vi "Autonomous Independent.vi"(5 "Servo Positions":T1, 7 "Auton Array":dbl[][](array[numeric])) -> (3 "LED ms toggle rate":u32=500)   [LabVIEW 2013]
doc: "This VI is called when autonomous begins, and will automatically be terminated when autonomous ends. You can carry out timed or sensor driven robot movement independently without needing to return to the caller."
uses:
  <vilib>/Rock Robotics/WPI/Relay/WPI_RelayValue.ctl
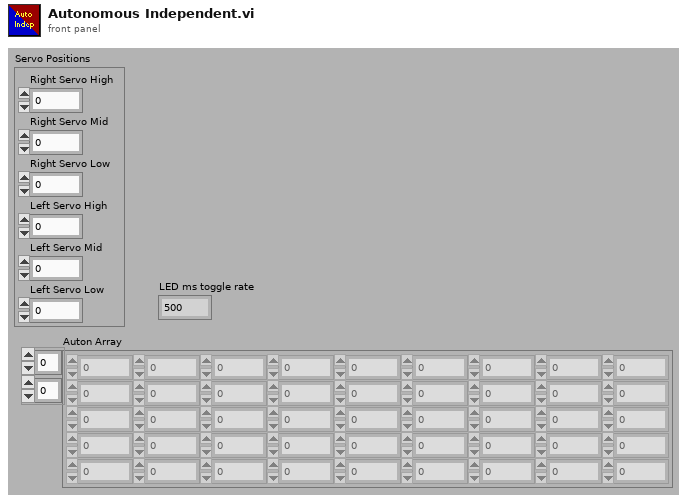
[diagram p1: front panel]
types:
  T1 = cluster{"Right Servo High":dbl, "Right Servo Mid":dbl, "Right Servo Low":dbl, "Left Servo High":dbl, "Left Servo Mid":dbl, "Left Servo Low":dbl}
  T2 = typedef "WPI_EncoderDevRef.ctl" = cluster{"DevStatus":errorcluster, "EncoderIndex":T3, "CounterIndex":T4, "DistancePerCount":dbl, "Decoding Type":T5}
  T3 = typedef "FPGA_EncoderIdx.ctl" = enum8{"Enc 0", "Enc 1", "Enc 2", "Enc 3", "Invalid"}
  T4 = typedef "FPGA_CounterCtrSystemIndex.ctl" = enum8{"Ctr 0", "Ctr 1", "Ctr 2", "Ctr 3", "Ctr 4", "Ctr 5", "Ctr 6", "Ctr 7", "Invalid"}
  T5 = typedef "WPI_EncoderType.ctl" = enum16{"1x", "2x", "4x"}
  T6 = typedef "WPI_GyroDevRef.ctl" = cluster{"DevStatus":errorcluster, "Analog Module":T7, "Analog Channel":T8, "Offset":dbl, "Gain (VoltsPerDegree/Second)":dbl}
  T7 = typedef "FPGA_TypedefAnalogModule.ctl" = enum16{"Analog Module 1", "Analog Module 2"}
  T8 = typedef "FPGA_AIChannel.ctl" = enum8{"AI 1", "AI 2", "AI 3", "AI 4", "AI 5", "AI 6", "AI 7", "AI 8", "Invalid"}
  T9 = typedef "WPI_RelayValue.ctl" = enum16{"Off", "On", "Forward", "Reverse"}
  T10 = typedef "WPI_RelayDevRef.ctl" = cluster{"DevStatus":errorcluster, "Relay Channel":T11, "Digital Module":T12, "Relay Direction":T13}
  T11 = typedef "FPGA_DIORelayChannel.ctl" = enum8{"Relay 1", "Relay 2", "Relay 3", "Relay 4", "Relay 5", "Relay 6", "Relay 7", "Relay 8", "Invalid"}
  T12 = typedef "FPGA_TypedefDigitalModule.ctl" = enum16{"Digital Module 1", "Digital Module 2"}
  T13 = typedef "WPI_RelayDirection.ctl" = enum16{"Both directions", "Forward only", "Reverse only"}
  T14 = typedef "WPI_MotorControlDeviceRef.ctl" = cluster{"DeviceStatus":errorcluster, "Type":enum16{"PWM", "CAN"}, "PWM":cluster{"Digital Module":T12, "PWM Channel":T15, "DeadBand":T16}, "CAN":cluster{"Device Number":u8, "Control Mode":T17, "Semaphore":T18, "Max Vout":dbl}, "Invert":bool, "TransformRef":T19, "InvTransformRef":T19}
  T15 = typedef "FPGA_DIOPWMChannel.ctl" = enum8{"PWM 1", "PWM 2", "PWM 3", "PWM 4", "PWM 5", "PWM 6", "PWM 7", "PWM 8", "PWM 9", "PWM 10", "Invalid"}
  T16 = typedef "WPI_PWMDeadband.ctl" = cluster{"Name":string, "maxPositivePwm":i32, "minPositivePwm":i32, "centerPwm":i32, "maxNegativePwm":i32, "minNegativePwm":i32, "angularRange":u16}
  T17 = typedef "WPI_CANJaguar_ControlMode.ctl" = enum8{"Percent VBus", "Current", "Speed", "Position", "Voltage"}
  T18 = typedef "Semaphore RefNum" = refnum<k1>
  T19 = typedef "WPI_PWMTransform_ConPane.ctl" = refnum<vi>
  T20 = typedef "WPI_ServoDeviceRef.ctl" = cluster{"DeviceStatus":errorcluster, "Digital Module":T12, "PWM Channel":T15, "DeadBand":T16}
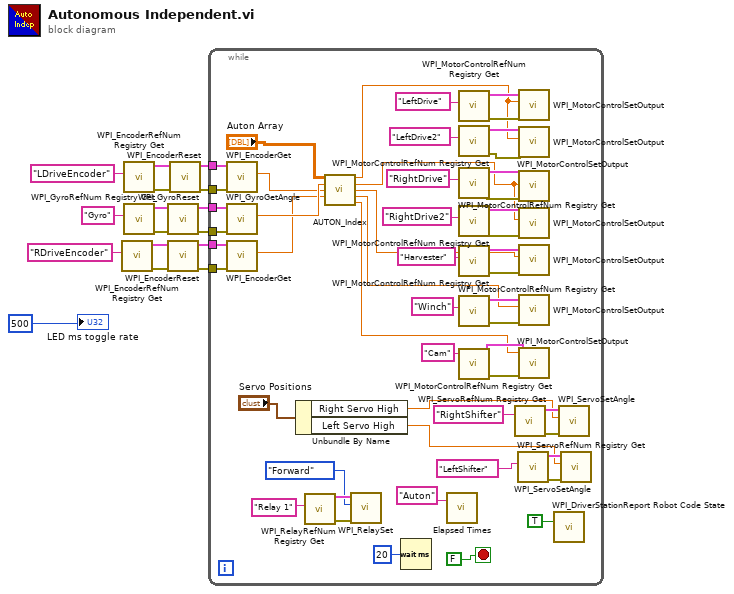
[diagram p0: block diagram]
diagram:
  n1 = call <vilib>:"WPI_EncoderRefNum Registry Get.vi"("refnum name"="RDriveEncoder") -> ("error out"=w3:errorcluster, "EncoderDevRef"=w5:T2)  [unwired: 9 in]
  n2 = call <vilib>:"WPI_EncoderRefNum Registry Get.vi"("refnum name"="LDriveEncoder") -> ("error out"=w9:errorcluster, "EncoderDevRef"=w8:T2)  [unwired: 9 in]
  n3 = call <vilib>:"WPI_GyroRefNum Registry Get.vi"("refnum name"="Gyro") -> ("error out"=w13:errorcluster, "GyroDevRef"=w14:T6)  [unwired: 9 in]
  n4 = call <vilib>:"WPI_GyroReset.vi"("error in (no error)"=w13, "GyroDevRef"=w14) -> ("error out"=w11:errorcluster, "GyroDevRef"=w12:T6)  [unwired: 8 in]
  n5 = call <vilib>:"WPI_EncoderReset.vi"("error in (no error)"=w3, "EncoderDevRef"=w5) -> ("error out"=w1:errorcluster, "EncoderDevRef"=w2:T2)  [unwired: 8 in]
  n6 = call <vilib>:"WPI_EncoderReset.vi"("error in (no error)"=w9, "EncoderDevRef"=w8) -> ("error out"=w6:errorcluster, "EncoderDevRef"=w7:T2)  [unwired: 8 in]
  n7 = while {
    tunnel: w12 -> [w65]
    tunnel: w11 -> [w64]
    tunnel: w7 -> [w63]
    tunnel: w6 -> [w62]
    tunnel: w2 -> [w55]
    tunnel: w1 -> [w54]
    stop <- FALSE stop-if-true
    n8 = call <vilib>:"WPI_EncoderGet.vi"("error in (no error)"=w62, "EncoderDevRef"=w63) -> ("Distance"=w61:dbl)  [unwired: 4 in, 5 out]
    n9 = call <vilib>:"WPI_GyroGetAngle.vi"("error in (no error)"=w64, "GyroDevRef"=w65) -> ("Angle"=w66:dbl)  [unwired: 6 in, 3 out]
    n10 = call <vilib>:"WPI_EncoderGet.vi"("error in (no error)"=w54, "EncoderDevRef"=w55) -> ("Distance"=w53:dbl)  [unwired: 4 in, 5 out]
    n11 = Unbundle By Name("Servo Positions") -> ("Right Servo High"=w43:dbl, "Left Servo High"=w42:dbl)
    n12 = call <vilib>:"WPI_RelayRefNum Registry Get.vi"("refnum name"="Relay 1") -> ("error out"=w57:errorcluster, "RelayDevRef"=w59:T10)  [unwired: 9 in]
    n13 = call "AUTON_Index.vi"("Auton Array"="Auton Array", "MeasuredHeading"=w66, "LeftEncoder"=w61, "RightEncoder"=w53) -> ("Right Drive"=w19:dbl, "Left Drive"=w20:dbl, "Harvester"=w29:dbl, "Winch"=w22:dbl, "Cam"=w21:dbl)  [unwired: 7 in]
    n14 = call <vilib>:"WPI_RelaySet.vi"("error in (no error)"=w57, "RelayValue"=WPI_RelayValue."Forward", "RelayDevRef"=w59) -> ()  [unwired: 7 in, 2 out]
    n15 = Wait (ms)(milliseconds to wait=u32 20) -> ()  [unwired: 1 out]
    n16 = call "Elapsed Times.vi"("Call Name"="Auton") -> ()  [unwired: 2 in, 1 out]
    n17 = call <vilib>:"WPI_MotorControlRefNum Registry Get.vi"("refnum name"="LeftDrive") -> ("error out"=w36:errorcluster, "MotorControlDevRef"=w39:T14)  [unwired: 9 in]
    n18 = call <vilib>:"WPI_MotorControlRefNum Registry Get.vi"("refnum name"="LeftDrive2") -> ("error out"=w37:errorcluster, "MotorControlDevRef"=w38:T14)  [unwired: 9 in]
    n19 = call <vilib>:"WPI_MotorControlRefNum Registry Get.vi"("refnum name"="RightDrive") -> ("error out"=w30:errorcluster, "MotorControlDevRef"=w31:T14)  [unwired: 9 in]
    n20 = call <vilib>:"WPI_MotorControlRefNum Registry Get.vi"("refnum name"="RightDrive2") -> ("error out"=w32:errorcluster, "MotorControlDevRef"=w33:T14)  [unwired: 9 in]
    n21 = call <vilib>:"WPI_MotorControlRefNum Registry Get.vi"("refnum name"="Harvester") -> ("error out"=w34:errorcluster, "MotorControlDevRef"=w35:T14)  [unwired: 9 in]
    n22 = call <vilib>:"WPI_MotorControlRefNum Registry Get.vi"("refnum name"="Winch") -> ("error out"=w28:errorcluster, "MotorControlDevRef"=w24:T14)  [unwired: 9 in]
    n23 = call <vilib>:"WPI_MotorControlRefNum Registry Get.vi"("refnum name"="Cam") -> ("error out"=w25:errorcluster, "MotorControlDevRef"=w23:T14)  [unwired: 9 in]
    n24 = call <vilib>:"WPI_ServoRefNum Registry Get.vi"("refnum name"="RightShifter") -> ("error out"=w46:errorcluster, "ServoDeviceRef"=w47:T20)  [unwired: 9 in]
    n25 = call <vilib>:"WPI_ServoRefNum Registry Get.vi"("refnum name"="LeftShifter") -> ("error out"=w48:errorcluster, "ServoDeviceRef"=w49:T20)  [unwired: 9 in]
    n26 = call <vilib>:"WPI_MotorControlSetOutput.vi"("error in (no error)"=w36, "Output"=w19, "MotorControlDevRef"=w39) -> ()  [unwired: 6 in, 3 out]
    n27 = call <vilib>:"WPI_MotorControlSetOutput.vi"("error in (no error)"=w37, "Output"=w19, "MotorControlDevRef"=w38) -> ()  [unwired: 6 in, 3 out]
    n28 = call <vilib>:"WPI_MotorControlSetOutput.vi"("error in (no error)"=w30, "Output"=w20, "MotorControlDevRef"=w31) -> ()  [unwired: 6 in, 3 out]
    n29 = call <vilib>:"WPI_MotorControlSetOutput.vi"("error in (no error)"=w32, "Output"=w20, "MotorControlDevRef"=w33) -> ()  [unwired: 6 in, 3 out]
    n30 = call <vilib>:"WPI_MotorControlSetOutput.vi"("error in (no error)"=w34, "Output"=w29, "MotorControlDevRef"=w35) -> ()  [unwired: 6 in, 3 out]
    n31 = call <vilib>:"WPI_MotorControlSetOutput.vi"("error in (no error)"=w28, "Output"=w22, "MotorControlDevRef"=w24) -> ()  [unwired: 6 in, 3 out]
    n32 = call <vilib>:"WPI_MotorControlSetOutput.vi"("error in (no error)"=w25, "Output"=w21, "MotorControlDevRef"=w23) -> ()  [unwired: 6 in, 3 out]
    n33 = call <vilib>:"WPI_DriverStationReport Robot Code State.vi"("Autonomous"=TRUE) -> ()  [unwired: 10 in, 1 out]
    n34 = call <vilib>:"WPI_ServoSetAngle.vi"("error in (no error)"=w46, "Angle"=w43, "ServoDeviceRef"=w47) -> ()  [unwired: 7 in, 2 out]
    n35 = call <vilib>:"WPI_ServoSetAngle.vi"("error in (no error)"=w48, "Angle"=w42, "ServoDeviceRef"=w49) -> ()  [unwired: 7 in, 2 out]
  }
  "LED ms toggle rate" <- u32 500 ("LED ms toggle rate")
